vi "Pickbufferbysize.vi"(9 "buffer size":u64, 10 "Buffers":T1[](array[typedef])) -> (1 "found":bool, 2 "buffer found":T1, 3 "index":i32)   [LabVIEW 2016]
uses:
  private/vis/BufferStruct.ctl
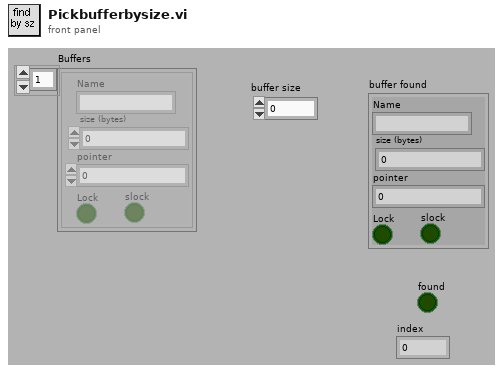
[diagram p1: front panel]
types:
  T1 = typedef "BufferStruct.ctl" = cluster{"Name":string, "size (bytes)":u64, "pointer":u64, "Lock":bool, "slock":bool}
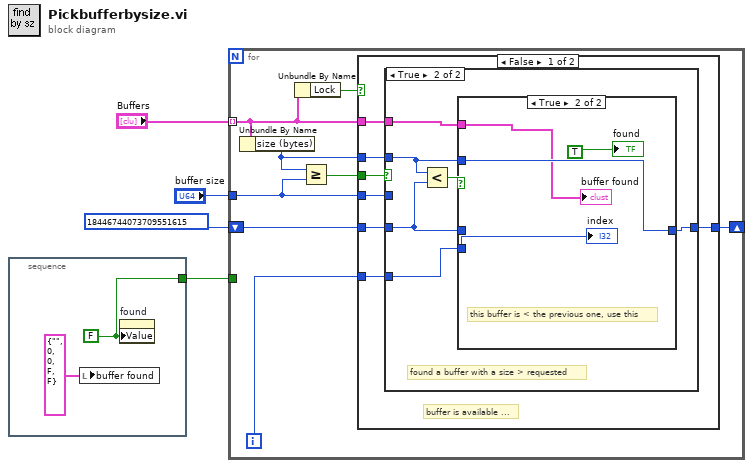
[diagram p0: block diagram]
diagram:
  n1 = stacked-sequence {
    tunnel: [w6] -> w1
    frame #0 {
      w6 = FALSE
      n2 = local write "buffer found"(T1 {"Name"="", "size (bytes)"=0, "pointer"=0, "Lock"=FALSE, "slock"=FALSE} ("buffer found")) -> ()
      n3 = property on="found" class="Bool (strict)"("Value"=w6) -> ()  [unwired: 2 in, 2 out]
    }
  }
  n4 = for {
    tunnel: "Buffers" -> [w8] mode=indexing
    tunnel: "buffer size" -> [w12]
    shift-right: [w9] -> _
    shift-left: u64 18446744073709551615 -> [w10]
    tunnel: w1 -> [_]
    i -> [w13]
    n5 = Unbundle By Name(w8) -> ("size (bytes)"=w11:u64)
    n6 = Unbundle By Name(w8) -> ("Lock"=w7:bool)
    n7 = Greater Or Equal?(x=w11, y=w12) -> (x >= y?=w14:bool)
    n8 = case shown="False" w7 {
      tunnel: w14 -> [w21 _]
      tunnel: w8 -> [w20 _]
      tunnel: w13 -> [w19 _]
      tunnel: w12 -> [w18 _]
      tunnel: w11 -> [w17 _]
      tunnel: w10 -> [w16 w34]
      tunnel: [w15 w34] -> w9
      frame False {
        # "buffer is available ..."
        n9 = case shown="True" w21 {
          tunnel: w20 -> [_ w23]
          tunnel: w19 -> [_ w27]
          tunnel: w18 -> [_ _]
          tunnel: w17 -> [_ w25]
          tunnel: w16 -> [w22 w24]
          tunnel: [w22 w26] -> w15
          frame False {
            # "buffer size < requested size: skip"
          }
          frame True {
            # "found a buffer with a size > requested"
            n10 = Less?(x=w25, y=w24) -> (x < y?=w28:bool)
            n11 = case shown="True" w28 {
              tunnel: w27 -> [_ w33]
              tunnel: [w29 w32] -> w26
              tunnel: w25 -> [_ w32]
              tunnel: w24 -> [w29 _]
              tunnel: w23 -> [_ w30]
              frame False {
                # "there is previous match which \nis better"
              }
              frame True {
                # "this buffer is < the previous one, use this"
                "index" <- w33
                "found" <- TRUE
                "buffer found" <- w30
              }
            }
          }
        }
      }
      frame True {
        # "buffer is locked, skip it"
      }
    }
  }
